vi "mxwScript_Cmnd2Str_setWireRoutingParameters.vi"(8 "error in (no error)":errorcluster, 11 "data":variant) -> (0 "error out":errorcluster, 3 "outputString":string)   [LabVIEW 2020]
uses:
  codeGenAPISupport.llb/cgAPI_mxwScript_Wire_RoutingParameters.ctl
  codeGenAPISupport.llb/cgAPI_mxwScript_Wire_RoutingAlgorithm.ctl
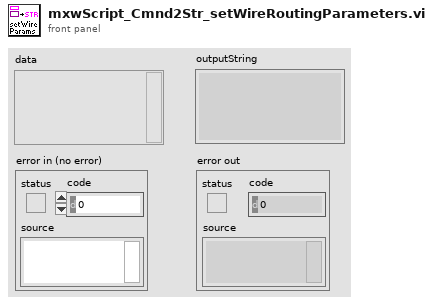
[diagram p1: front panel]
types:
  T1 = typedef "cgAPI_mxwScript_Wire_RoutingParameters.ctl" = cluster{"routingAlgorithm":T2, "offset":i32, "AIWeights":cluster{"edgeCrossing":i32, "wireKink":i32, "wireCrossing":i32, "lengthPerPixel":i32}}
  T2 = typedef "cgAPI_mxwScript_Wire_RoutingAlgorithm.ctl" = enum16{"None", "LV", "AI"}
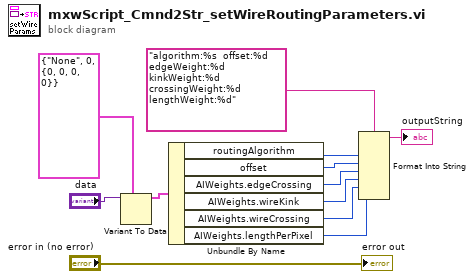
[diagram p0: block diagram]
diagram:
  n1 = Variant To Data(type=T1 {"routingAlgorithm"=enum."None", "offset"=0, "AIWeights"={"edgeCrossing"=0, "wireKink"=0, "wireCrossing"=0, "lengthPerPixel"=0}} ("wireRoutingParameters"), Variant="data") -> (data=w10:T1)  [unwired: 1 in, 1 out]
  n2 = Unbundle By Name(w10) -> ("routingAlgorithm"=w6:T2, "offset"=w5:i32, "AIWeights.edgeCrossing"=w4:i32, "AIWeights.wireKink"=w2:i32, "AIWeights.wireCrossing"=w1:i32, "AIWeights.lengthPerPixel"=w3:i32)
  n3 = Format Into String(format string="algorithm:%s  offset:%d  edgeWeight:%d  kinkWeight:%d  crossingWeight:%d  lengthWeight:%d", w6, w5, w4, w2, w1, w3) -> (resulting string=→"outputString":string)  [unwired: 2 in, 1 out]
  "error out" <- "error in (no error)"
